vi "pume_write.vi"() -> ()   [LabVIEW 2013]
uses:
  SubVI/NI Modbus.llb/MB Serial Master Query Write Single Register (poly).vi
panel:
  in  "Boolean":bool=TRUE
  in  "Register":u8=128 format="%x"
  in  "Address":u16=9600
  in  "Serial Parameters":T1={"Mode"=enum."RTU", "Slave Address"=1} {"Slave Address" format="%x"}
  in  "Timeout":u32=10000
  in  "Flow Control":u16(ring) items=["None", "XON/XOFF", "RTS/CTS", "XON/XOFF & RTS/CTS", "DTR/DSR", "XON/XOFF & DTR/DSR"]
  in  "Parity":u16(ring) items=["None", "Odd", "Even", "Mark", "Space"]
  in  "Baud Rate":u32=9600
  in  "Port":refnum<visa-resource-name>
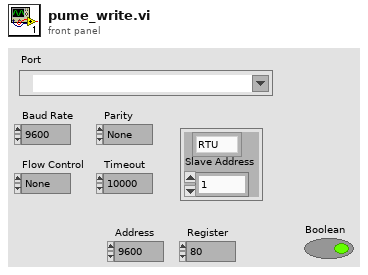
[diagram p1: front panel]
types:
  T1 = cluster{"Mode":enum16{"RTU", "ASCII"}, "Slave Address":u8}
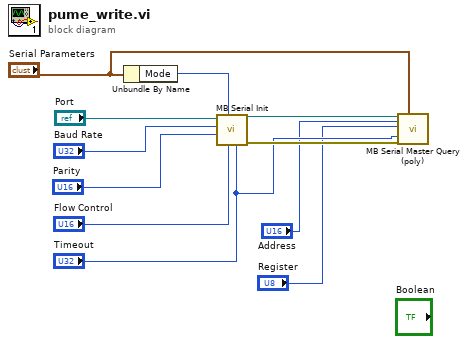
[diagram p0: block diagram]
diagram:
  n1 = Unbundle By Name("Serial Parameters") -> ("Mode"=w7:enum16{"RTU", "ASCII"})
  n2 = call "MB Serial Init.vi"("Timeout"="Timeout", "Flow Control"="Flow Control", "Mode"=w7, "Parity"="Parity", "Baud Rate"="Baud Rate", "VISA resource name"="Port") -> ("error out"=w4:errorcluster, "VISA resource name out"=w5:refnum<visa-resource-name>)  [unwired: 1 in, 3 out]
  n3 = call-poly "MB Serial Master Query (poly).vi"("VISA resource name"=w5, "Address"="Address", "Holding Register"="Register", "Timeout"="Timeout", "error in"=w4, "Serial Parameters"="Serial Parameters") -> ()  [unwired: 11 in, 3 out]
